vi "Transfer Images Data to UI New.vi"(0 "fpga interface in":refnum<k20>, 1 "'stop' notifier":refnum<notifier>, 3 "measure call context in":refnum<class "Measure Call Context.lvclass">, 5 "Active Channel":string[](array[string]), 11 "error in":errorcluster, 12 "References":T1, 13 "raw display notifier":refnum<notifier>) -> (4 "fpga interface out":refnum<k20>, 15 "error out":errorcluster)   [LabVIEW 2026]
doc: "Handles frame grabbing, and prepare data for sendig it to the UI."
uses:
  <vilib>/Plug-In SDKs/Measurements/Measure Call Context/Measure Call Context.lvclass
  deps/NI148X/Getting Started/Host/Common/Types/Serial Channel Display Parameters.ctl
  <vilib>/vision/Image Controls.llb/IMAQ Image.ctl
  deps/NI148X/Getting Started/Host/Common/Types/RAW Interpretation for Display.ctl
  ttashjia/GSE/Host/Common/Types/148x_Common_FPGA_Reference.ctl
  <instrlib>/FlexRIO/CSI-2/v2/Common/Types/LLP Data Type.ctl
  Measurement Results.ctl
  <vilib>/Utility/error.llb/Error Cluster From Error Code.vi
  <vilib>/rvi/errors/niLvFpgaAdjustHostInterfaceError.vi
  <vilib>/rvi/interface/nirviReadWriteControl/nirviReadWriteControl.xnode
  Automotive Vision.lvclass/Automotive Vision.ctl
  deps/NI148X/Getting Started/Host/Common/GettingStarted_Common_148X_Host.lvlib
  <instrlib>/FlexRIO/CSI-2/v2/Common/NI CSI-2 API Common v2.lvlib
  Automotive Vision.lvclass
  Automotive-Vision OOB Data Transfer/Automotive-Vision OOB Data Transfer.lvlib
  NiFpgaLv.dll
  <vilib>/rvi/interface/Simulation/niFpgaSimulationCallBeginRW.vi
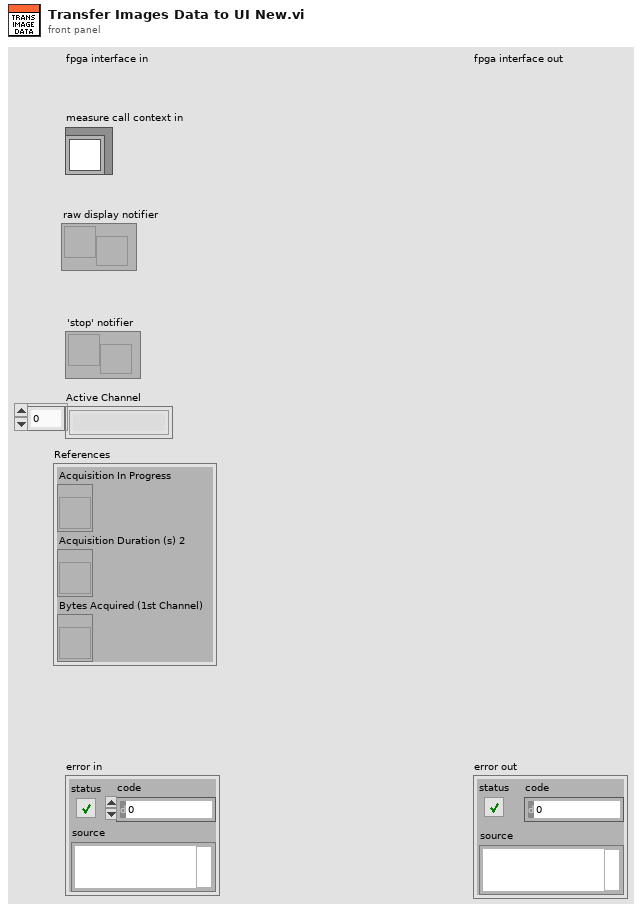
[diagram p1: front panel]
types:
  T1 = cluster{"Acquisition In Progress":refnum<vi>, "Acquisition Duration (s) 2":refnum<vi>, "Bytes Acquired (1st Channel)":refnum<vi>}
  T2 = typedef "NI CSI-2 API Common v2.lvlib/LLP Data Type.ctl" = enum8{"Frame Start", "Frame End", "Line Start", "Line End", "End of Transmission", "Reserved 0", "Reserved 1", "Reserved 2", "Generic Short Packet 1", "Generic Short Packet 2", "Generic Short Packet 3", "Generic Short Packet 4", "Generic Short Packet 5", "Generic Short Packet 6", "Generic Short Packet 7", "Generic Short Packet 8", "Null", "Blanking Data", "Embedded 8-bit non Image Data", "Generic Long Packet 1", "Generic Long Packet 2", "Generic Long Packet 3", "Generic Long Packet 4", "Reserved 3", "YUV420 8-bit", "YUV420 10-bit", "Legacy YUV420 8-bit", "Reserved 4", "YUV420 8-bit Chroma Shifted", "YUV420 10-bit Chroma Shifted", "YUV422 8-bit", "YUV422 10-bit", "RGB444", "RGB555", "RGB565", "RGB666", "RGB888", "Reserved 5", "Reserved 6", "RAW 24", "RAW 6", "RAW 7", "RAW 8", "RAW 10", "RAW 12", "RAW 14", "RAW 16", "RAW 20", "User Defined 8-bit Data 1", "User Defined 8-bit Data 2", "User Defined 8-bit Data 3", "User Defined 8-bit Data 4", "User Defined 8-bit Data 5", "User Defined 8-bit Data 6", "User Defined 8-bit Data 7", "User Defined 8-bit Data 8", "USL Command", "Reserved 7", "Reserved 8", "Reserved 9", "Reserved 10", "Reserved 11", "Reserved 12", "LRTE EPD Spacer"}
  T3 = cluster{"serial channel":fxp<+,3,3>, "frame number":u16, "data type":T2, "width":u16, "height":u16, "image bytes":u32, "total bytes":u32, "little endian":bool, "Status":string}
  T4 = typedef "148x_Common_FPGA_Reference.ctl" = refnum<k20>
  T5 = typedef "GettingStarted_Common_148X_Host.lvlib/Serial Channel Display Parameters.ctl" = cluster{"images":cluster{"grayscale":T6, "color":T6}, "RAW parameters":cluster{"interpretation":T7, "bayer parameters":cluster{"pattern":i32, "algorithm":i32, "red gain":dbl, "green gain":dbl, "blue gain":dbl}}}
  T6 = typedef "IMAQ Image.ctl" = refnum<image>
  T7 = typedef "GettingStarted_Common_148X_Host.lvlib/RAW Interpretation for Display.ctl" = enum16{"Grayscale", "Bayer", "RGB", "YUV422", "YUV420", "Legacy YUV420"}
  T8 = typedef "GettingStarted_Common_148X_FPGA.lvlib/Image Metadata.ctl" = cluster{"serial channel":fxp<+,3,3>, "frame number":u16, "data type":T2, "width":u16, "height":u16, "image bytes":u32, "total bytes":u32, "little endian":bool}
  T9 = typedef "Automotive-Vision OOB Data Transfer.lvlib/OOB to Logic Data.ctl" = cluster{"PauseResume":bool, "ExportPath":string, "ExportType":u16, "Export":bool}
  T10 = typedef "Automotive Vision.lvclass/Measurement Results.ctl" = cluster{"ACQ. IN PROGRESS":bool, "IMAGE PIXEL DATA":u32[], "ACQ. DURATION (s)":dbl, "SOURCE RATE (fps)":dbl, "BYTES ACQUIRED":u64, "FRAME COUNT":u64, "POC VOLTAGE (V)":dbl, "POC CURRENT (A)":dbl, "ERROR":bool, "STATE MESSAGE":string, "IMAGE DATA":string, "OOB gRPC Port":i32, "HEIGHT":u64, "WIDTH":u64}
  T11 = cluster{"image pixel data fifo overflow":bool, "image metadata fifo overflow":bool}[]
  T12 = cluster{"image pixel data fifo overflow":bool, "image metadata fifo overflow":bool}
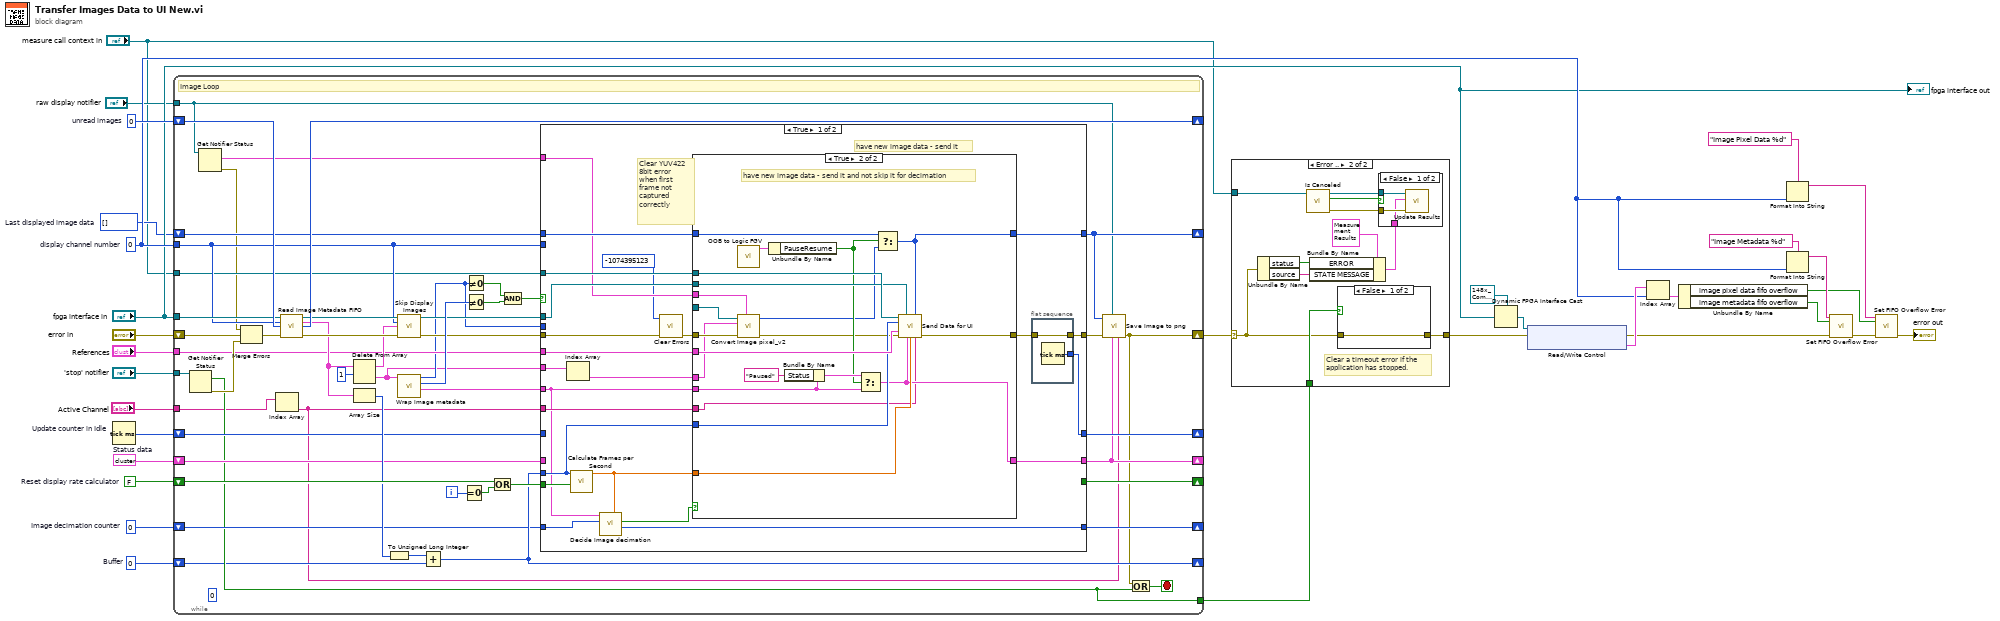
[diagram p0: block diagram]
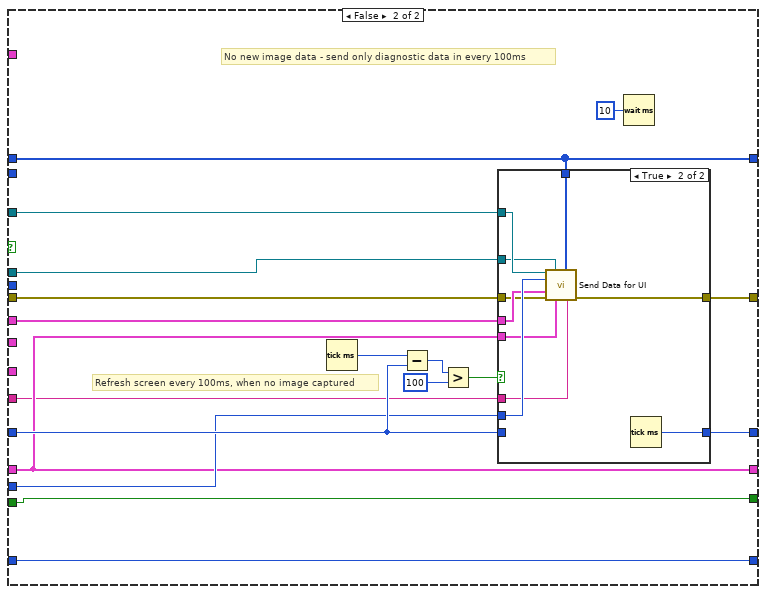
[diagram p3: hidden frame]
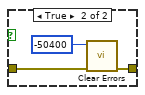
[diagram p7: hidden frame]
diagram:
  w4 = T3 {"serial channel"=0.0, "frame number"=0, "data type"=enum."Frame Start", "width"=0, "height"=0, "image bytes"=0, "total bytes"=0, "little endian"=FALSE, "Status"="Ready for Acquisition"}  # Status data
  w22 = 0  # display channel number
  w7 = u32 0  # Image decimation counter
  w8 = u32[] []  # Last displayed image data
  w14 = u32 0  # Buffer
  w15 = FALSE  # Reset display rate calculator
  w31 = u32 0  # unread images
  n1 = Tick Count (ms) "Update counter in Idle"() -> (millisecond timer value=w9:u32)
  n2 = while {
    shift-right: [w38] -> w13
    shift-left: "error in" -> [w56]
    tunnel: "fpga interface in" -> [w59]
    shift-right: [w79] -> _
    shift-left: w31 -> [w70]
    tunnel: w22 -> [w55]
    shift-right: [w74] -> _
    shift-left: w15 -> [w71]
    shift-right: [w61] -> _
    shift-left: w14 -> [w42]
    tunnel: [w44] -> w11
    tunnel: "'stop' notifier" -> [w58]
    shift-right: [w53] -> _
    shift-left: w9 -> [w54]
    shift-right: [w41] -> _
    shift-left: w8 -> [w52]
    shift-right: [w50] -> _
    shift-left: w7 -> [w51]
    tunnel: "References" -> [w49]
    tunnel: "measure call context in" -> [w48]
    shift-right: [w39] -> _
    shift-left: w4 -> [w47]
    tunnel: "raw display notifier" -> [w35]
    tunnel: "Active Channel" -> [w37]
    i -> [w78]
    stop <- w80 stop-if-true
    (unwired) 0 ("index")
    # "Image Loop"
    n3 = Get Notifier Status(notifier=w58) -> (current notification=w44:bool, error out=w81:errorcluster)  [unwired: 1 in, 3 out]
    n4 = Get Notifier Status(notifier=w35) -> (current notification=w33:T5[], error out=w34:errorcluster)  [unwired: 1 in, 3 out]
    n5 = Merge Errors(w34, w56, w81) -> (w57:errorcluster)
    n6 = Index Array(array=w37) -> (element=w36:string)  [unwired: 1 in]
    n7 = call "Read Image Metadata FIFO.vi"("fpga inteface in"=w59, "display channel number"=w55, "number of images"=w70, "error in (no error)"=w57) -> ("fpga interface out"=w67:refnum<k20>, "image metadata"=w60:T8[], "images remaining"=w79:u32, "error out"=w64:errorcluster)  [unwired: 8 in]
    n8 = Delete From Array(array=w60, length=1) -> (deleted portion=w32:T8[], array with subset deleted=w63:T8[])  [unwired: 1 in]
    n9 = Array Size(array=w60) -> (size(s)=w62:i32)
    n10 = To Unsigned Long Integer(number=w62) -> (unsigned 32bit integer=w43:u32)
    n11 = call "Skip Display Images.vi"("fpga interface in"=w67, "display channel number"=w55, "image metadata"=w63, "error in (no error)"=w64) -> ("fpga interface out"=w66:refnum<k20>, "error out"=w65:errorcluster)  [unwired: 10 in]
    n12 = call "Wrap Image metadata.vi"("image metadata"=w32) -> ("element"=w46:T3, "Numeric"=w69:i32, "total bytes"=w45:u32)  [unwired: 8 in]
    n13 = Add(x=w43, y=w42) -> (x+y=w61:u32)
    n14 = Equal To 0?(x=w78) -> (x = 0?=w72:bool)
    n15 = Not Equal To 0?(x=w45) -> (x != 0?=w76:bool)
    n16 = Not Equal To 0?(x=w69) -> (x != 0?=w77:bool)
    n17 = Compound Arithmetic op=OR(w71, w72) -> (w73:bool)
    n18 = Compound Arithmetic op=AND(w76, w77) -> (w75:bool)
    n19 = case shown="True" w75 {
      tunnel: w65 -> [w90 w133]
      tunnel: w66 -> [w89 w131]
      tunnel: w55 -> [_ _]
      tunnel: [w102 w140] -> w40
      tunnel: w73 -> [w93 w147]
      tunnel: [_ w147] -> w74
      tunnel: w61 -> [w99 w137]
      tunnel: w45 -> [_ _]
      tunnel: w46 -> [w85 _]
      tunnel: w48 -> [w104 w134]
      tunnel: w49 -> [w103 w148]
      tunnel: w54 -> [_ w139]
      tunnel: [w101 w141] -> w53
      tunnel: w52 -> [w98 w138]
      tunnel: [w100 w138] -> w41
      tunnel: w51 -> [w97 w136]
      tunnel: [w96 w136] -> w50
      tunnel: w47 -> [_ w135]
      tunnel: [w94 w135] -> w39
      tunnel: w36 -> [w92 w132]
      tunnel: w33 -> [w86 _]
      tunnel: w32 -> [w88 _]
      frame True {
        # "Clear YUV422 8bit error when first frame not captured correctly"
        # "have new image data - send it"
        n20 = Index Array(array=w88) -> (element=w87:T8)  [unwired: 1 in]
        n21 = call <vilib>:"Calculate Frames per Second.vi"("Reset"=w93, "Buffer Number"=w99) -> ("Acquired Frames/s"=w84:dbl)  [unwired: 7 in, 2 out]
        n22 = call "Decide Image decimation.vi"("FPS"=w84, "Image decimation counter in"=w97, "element in"=w85) -> ("Image decimation counter out"=w96:u32, "send current image data"=w95:bool)  [unwired: 7 in]
        n23 = call <vilib>:"Clear Errors.vi"("error in (no error)"=w90, "specific error code to clear (0: all)"=-1074395123) -> ("error out"=w82:errorcluster)  [unwired: 4 in, 1 out]
        n24 = case shown="True" w95 {
          tunnel: [w105 w120] -> w91
          tunnel: w84 -> [_ w128]
          tunnel: w85 -> [w106 w115]
          tunnel: w104 -> [_ w127]
          tunnel: w103 -> [_ w126]
          tunnel: [w107 w125] -> w100
          tunnel: w99 -> [_ w124]
          tunnel: w98 -> [w107 w123]
          tunnel: [w106 w122] -> w94
          tunnel: w89 -> [_ w121]
          tunnel: w92 -> [_ w114]
          tunnel: w82 -> [w105 w113]
          tunnel: _ -> [_ w111]
          tunnel: w87 -> [_ w109]
          tunnel: w86 -> [_ w108]
          frame False {
            # "have new image data - but skip the sending to not overload UI with data transfer"
          }
          frame True {
            # "have new image data - send it and not skip it for decimation"
            n25 = call "OOB to Logic FGV.vi"() -> ("OOB to Logic Data out"=w117:T9)  [unwired: 10 in, 1 out]
            n26 = call "Convert Image pixel_v2.vi"("serial channel display parameters"=w108, "error in"=w113, "image metadata"=w109, "Refnum in"=w111) -> ("error out"=w112:errorcluster, "Image Pixels (U32)"=w110:u32[])  [unwired: 6 in]
            n27 = Unbundle By Name(w117) -> ("PauseResume"=w116:bool)
            n28 = Bundle By Name(cluster=w115, "Status"="Paused") -> (w119:T3)
            n29 = Select(t=w119, s=w116, f=w115) -> (s? t:f=w122:T3)
            n30 = Select(t=w123, s=w116, f=w110) -> (s? t:f=w125:u32[])
            n31 = call "Send Data for UI.vi"("Measure Call Context in"=w127, "fpga interface in"=w121, "Last displayed image data"=w125, "FrameCount"=w124, "References"=w126, "error in"=w112, "Status data"=w122, "SOURCE RATE (fps)"=w128, "Active Channel"=w114) -> ("error out"=w120:errorcluster)  [unwired: 6 in]
          }
        }
        n32 = flat-sequence {
          tunnel: [w130] -> w102
          tunnel: w91 -> [w130]
          tunnel: [w129] -> w101
          frame #0 {
            n33 = Tick Count (ms)() -> (millisecond timer value=w129:u32)
          }
        }
      }
      frame False {
        # "Refresh screen every 100ms, when no image captured"
        # "No new image data - send only diagnostic data in every 100ms"
        n34 = Tick Count (ms)() -> (millisecond timer value=w145:u32)
        n35 = Subtract(x=w145, y=w139) -> (x-y=w144:u32)
        n36 = Greater?(x=w144, y=u32 100) -> (0:w142:bool)
        n37 = case shown="True" w142 {
          tunnel: w133 -> [w150 w153]
          tunnel: [w150 w160] -> w140
          tunnel: w135 -> [_ w155]
          tunnel: w148 -> [_ w156]
          tunnel: [w149 w159] -> w141
          tunnel: w139 -> [w149 _]
          tunnel: w138 -> [_ w158]
          tunnel: w137 -> [_ w157]
          tunnel: w134 -> [_ w154]
          tunnel: w132 -> [_ w152]
          tunnel: w131 -> [_ w151]
          frame False {
          }
          frame True {
            n38 = call "Send Data for UI.vi"("Measure Call Context in"=w154, "fpga interface in"=w151, "Last displayed image data"=w158, "FrameCount"=w157, "References"=w156, "error in"=w153, "Status data"=w155, "Active Channel"=w152) -> ("error out"=w160:errorcluster)  [unwired: 7 in]
            n39 = Tick Count (ms)() -> (millisecond timer value=w159:u32)
          }
        }
        n40 = Wait (ms)(milliseconds to wait=u32 10) -> ()  [unwired: 1 out]
      }
    }
    n41 = call "Save Image to png.vi"("Channel"=w36, "image metadata"=w39, "raw display notifier"=w35, "error in"=w40, "Last displayed image data"=w41) -> ("error out"=w38:errorcluster)  [unwired: 6 in]
    n42 = Compound Arithmetic op=OR(w38, w44) -> (w80:bool)
  }
  n43 = case shown="Error .." w13 {
    selector: w13 -> [w161 w165]
    tunnel: [w161 w172] -> w26
    tunnel: w11 -> [_ w171]
    tunnel: "measure call context in" -> [_ w162]
    frame No Error {
    }
    frame Error {
      # "Clear a timeout error if the application has stopped."
      n44 = Unbundle By Name(w165) -> ("status"=w164:bool, "source"=w163:string)
      n45 = call <vilib>:"Is Canceled.vi"("measure call context in"=w162) -> ("error out"=w169:errorcluster, "is canceled?"=w168:bool, "measure call context out"=w170:refnum<class "Measure Call Context.lvclass">)  [unwired: 8 in]
      n46 = Bundle By Name(cluster=T10 {"ACQ. IN PROGRESS"=FALSE, "IMAGE PIXEL DATA"=[], "ACQ. DURATION (s)"=0.0, "SOURCE RATE (fps)"=0.0, "BYTES ACQUIRED"=0, "FRAME COUNT"=0, "POC VOLTAGE (V)"=0.0, "POC CURRENT (A)"=0.0, "ERROR"=FALSE, "STATE MESSAGE"="", "IMAGE DATA"="", "OOB gRPC Port"=0, "HEIGHT"=0, "WIDTH"=0} ("Measurement Results"), "ERROR"=w164, "STATE MESSAGE"=w163) -> (w166:T10)
      n47 = case shown="False" w171 {
        tunnel: w165 -> [w176 w179]
        tunnel: [w176 w177] -> w172
        frame False {
        }
        frame True {
          n48 = call <vilib>:"Clear Errors.vi"("error in (no error)"=w179, "specific error code to clear (0: all)"=-50400 ("y")) -> ("error out"=w177:errorcluster)  [unwired: 4 in, 1 out]
        }
      }
      n49 = case shown="False" w168 {
        tunnel: w170 -> [w175 _]
        tunnel: w169 -> [w174 _]
        tunnel: w166 -> [w173 _]
        frame False {
          n50 = call <vilib>:"Update Results.vi"("error in"=w174, "measurement results"=w173, "measure call context in"=w175) -> ()  [unwired: 7 in, 2 out]
        }
        frame True {
        }
      }
    }
  }
  n51 = Dynamic FPGA Interface Cast(Session In=T4 refnum ("FPGA VI Reference Out"), Type="fpga interface in") -> (Session Out=w27:T4)
  n52 = xnode ("Read/Write Control")("FPGA VI Reference In"=w27, "error in"=w26) -> ("error out"=w25:errorcluster, "display channel status"=w29:T11)  [unwired: 1 out]
  n53 = Index Array(array=w29, index=w22) -> (element=w30:T12)
  n54 = Unbundle By Name(w30) -> ("image pixel data fifo overflow"=w17:bool, "image metadata fifo overflow"=w16:bool)
  n55 = Format Into String(format string="Image Pixel Data %d", w22) -> (resulting string=w19:string)  [unwired: 2 in, 1 out]
  n56 = Format Into String(format string="Image Metadata %d", w22) -> (resulting string=w18:string)  [unwired: 2 in, 1 out]
  n57 = call "Set FIFO Overflow Error.vi"("fifo name"=w18, "overflow"=w16, "error in (no error)"=w25) -> ("error out"=w21:errorcluster)  [unwired: 12 in]
  n58 = call "Set FIFO Overflow Error.vi"("fifo name"=w19, "overflow"=w17, "error in (no error)"=w21) -> ("error out"=→"error out":errorcluster)  [unwired: 12 in]
  "fpga interface out" <- "fpga interface in"
